vi "Control_Loop_Main.vi"(8 "error in (no error)":errorcluster) -> (0 "error out":errorcluster, 2 "loop":i32, 3 "pkg recived":timestamp)   [LabVIEW 2019, in "Service.lvlib"]
uses:
  Service.lvlib
  TypeDef/Control_loop_states.ctl
  TypeDef/AppData.ctl
  MsgQ/TypeDefs/CommandsQ.ctl
  MsgQ/TypeDefs/MsgQ_Commands.ctl
  zmq_multipart_lib/src_LabVIEW/zmq_mulipart_lib/zmq_multipart_lib.lvclass
  <vilib>/Field R&D Services/Logger/Type Definitions/Severity.ctl
  <vilib>/Field R&D Services/Logger/Support/Manager.vi
  <vilib>/Field R&D Services/Logger/Field_RnD_Services_Logger_Toolkit.lvlib
  mmw_command_lib/src_LabVIEW/mmW_commands/mmW_commands.lvlib
  MsgQ/MsgQ.lvlib
panel:
  out "status":T1
  out "data DVR out":refnum<data-value>
  out "Mode":enum16{"RF", "IF", "BB"}(ring)
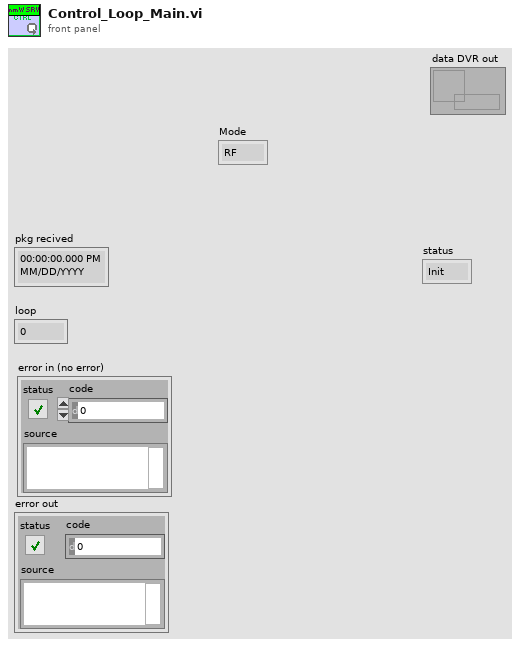
[diagram p1: front panel]
types:
  T1 = typedef "Service.lvlib/Control_loop_states.ctl" = enum16{"Init", "Create_listener", "Read", "Waiting_for_UI", "Send_response", "Close"}
  T2 = typedef "Service.lvlib/AppData.ctl" = cluster{"MsgQ":refnum<queue>, "Stop?":bool, "zmq sessions":cluster{"Control_endpoint":string, "Instr_endpoint":string}, "control-loop":cluster{"fromUI-Q":refnum<queue>, "toUI":refnum<user-event>, "Control_endpoint":string}, "UI-loop":cluster{"evnt_ref":refnum<event-registration>}, "logging":cluster{"level":dbl, "verbosity":dbl, "path":string, "Listener_ID":string}, "general_settings":cluster{"mmW_instr_ini_path":string, "mmW_instr_pid_path":string}}
  T3 = typedef "Field_RnD_Services_Logger_Toolkit.lvlib/Severity.ctl" = enum16{"Benign", "Warning", "Recoverable", "Fatal"}
  T4 = typedef "mmW_commands.lvlib/mode.ctl" = enum16{"RF", "IF", "BB"}
  T5 = typedef "mmW_commands.lvlib/commands.ctl" = enum16{"configure_fs", "configure_rf", "configure_trigger", "equalization_enable", "equalization_start", "lo_sync_enable", "equalization_stop", "get_instrument_status", "get_versions", "initialize_hw", "pop_rx", "set_log_level", "Shutdown", "start", "start_instrument_app", "stop", "trans", "transceive", "trigger_burst", "trigger_sync_enable", "Write TX", "resp_generic", "resp_waveform", "send_trigger", "fetch", "transceive2"}
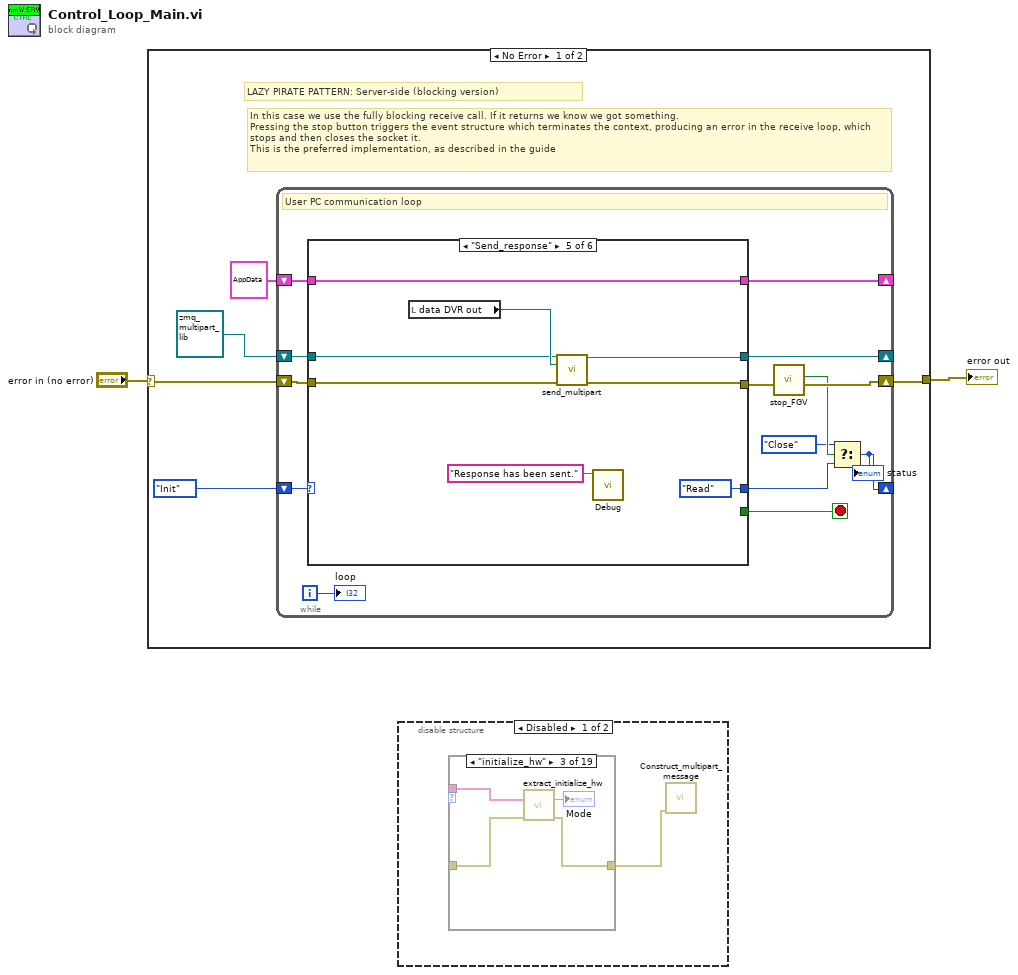
[diagram p0: block diagram]
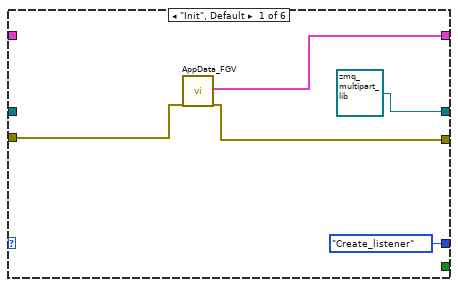
[diagram p2: hidden frame]
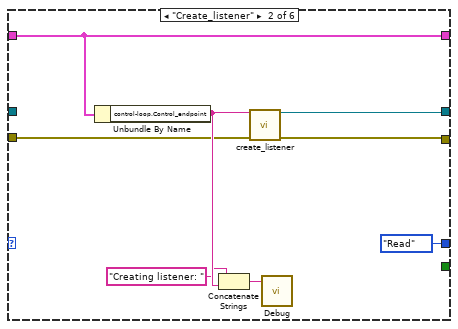
[diagram p3: hidden frame]
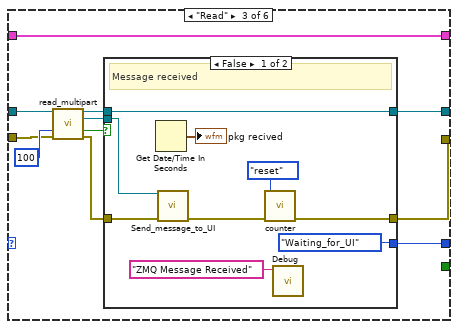
[diagram p4: hidden frame]
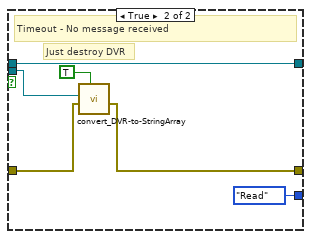
[diagram p5: hidden frame]
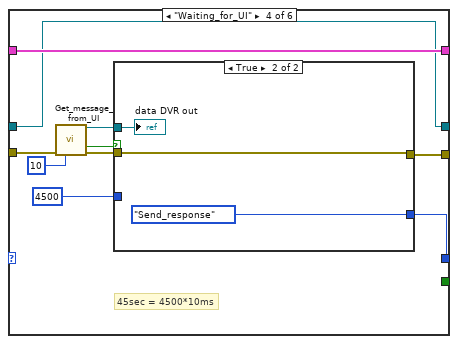
[diagram p6: hidden frame]
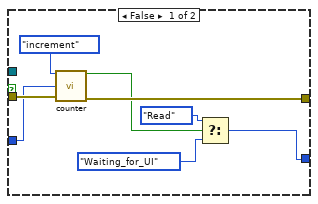
[diagram p7: hidden frame]
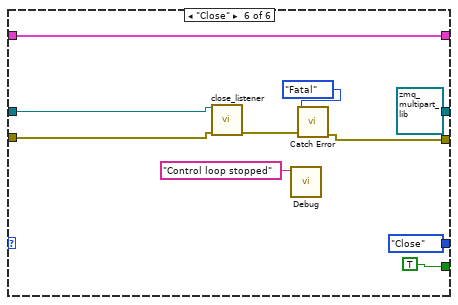
[diagram p8: hidden frame]
diagram:
  n1 = case shown="No Error" "error in (no error)" {
    selector: "error in (no error)" -> [w4 w100]
    tunnel: [w3 w100] -> w2
    frame No Error {
      # "In this case we use the fully blocking receive call. If it returns we know we got something.\nPressing the stop button triggers the event structure which terminates the context, producing an error in the receive loop, which stops and then closes the socket it.\nThis is the preferred implementation, as described in the guide"
      # "LAZY PIRATE PATTERN: Server-side (blocking version)"
      n2 = while {
        shift-right: [w19] -> w3
        shift-left: w4 -> [w17]
        shift-right: [w9] -> _
        shift-left: Control_loop_states."Init" -> [w15]
        shift-right: [w14] -> _
        shift-left: T2 {"MsgQ"=refnum, "Stop?"=FALSE, "zmq sessions"={"Control_endpoint"="", "Instr_endpoint"=""}, "control-loop"={"fromUI-Q"=refnum, "toUI"=refnum, "Control_endpoint"=""}, "UI-loop"={"evnt_ref"=refnum}, "logging"={"level"=0.0, "verbosity"=0.0, "path"="", "Listener_ID"=""}, "general_settings"={"mmW_instr_ini_path"="", "mmW_instr_pid_path"=""}} ("AppData out") -> [w13]
        shift-right: [w16] -> _
        shift-left: refnum<class "zmq_multipart_lib.lvclass"> refnum ("zmq_mlt out") -> [w18]
        i -> [w21]
        stop <- w12 stop-if-true
        # "User PC communication loop"
        n3 = case shown="\"Send_response\"" w15 {
          tunnel: [w24 w28 w45 w63 w84 w92] -> w20
          tunnel: w18 -> [_ _ w44 w61 w87 w90]
          tunnel: w17 -> [w25 w30 w42 w69 w85 w91]
          tunnel: [refnum<class "zmq_multipart_lib.lvclass"> refnum ("zmq_mlt out") w31 w37 w61 w86 refnum<class "zmq_multipart_lib.lvclass"> refnum ("zmq_mlt out")] -> w16
          tunnel: [w26 w29 w36 w70 w89 w99] -> w14
          tunnel: w13 -> [_ w29 w36 w70 w89 w99]
          tunnel: [Control_loop_states."Create_listener" Control_loop_states."Read" w35 w65 Control_loop_states."Read" Control_loop_states."Close"] -> w10
          tunnel: [_ _ _ _ _ TRUE] -> w12
          frame "Init", Default {
            n4 = call "AppData_FGV.vi"("error in (no error)"=w25) -> ("AppData out"=w26:T2, "error out"=w24:errorcluster)  [unwired: 17 in]
          }
          frame "Create_listener" {
            n5 = Unbundle By Name(w29) -> ("control-loop.Control_endpoint"=w34:string)
            n6 = Concatenate Strings("Creating listener: " ("string"), w34) -> (w33:string)
            n7 = call "create_listener.vi"("control_endpoint"=w34, "error in (no error)"=w30) -> ("zmq_mlt out"=w31:refnum<class "zmq_multipart_lib.lvclass">, "error out"=w28:errorcluster)  [unwired: 12 in]
            n8 = call <vilib>:"Debug.vi"("Message"=w33) -> ()  [unwired: 10 in, 1 out]
          }
          frame "Read" {
            n9 = call "read_multipart.vi"("zmq_mlt in"=w44, "timeout (ms)"=u32 100, "error in (no error)"=w42) -> ("zmq_mlt out"=w38:refnum<class "zmq_multipart_lib.lvclass">, "multipart message DVR"=w41:refnum<data-value>, "timeout?"=w40:bool, "error out"=w39:errorcluster)  [unwired: 8 in, 1 out]
            n10 = case shown="False" w40 {
              tunnel: w41 -> [w52 w59]
              tunnel: w39 -> [w51 w58]
              tunnel: [w46 w57] -> w45
              tunnel: w38 -> [w49 w60]
              tunnel: [w49 w60] -> w37
              tunnel: [Control_loop_states."Waiting_for_UI" Control_loop_states."Read"] -> w35
              frame False {
                # "Message received"
                n11 = Get Date/Time In Seconds() -> (seconds since 1Jan1904=→"pkg recived":timestamp)
                n12 = call "Send_message_to_UI.vi"("Data Value Reference in"=w52, "error in (no error)"=w51) -> ("error out"=w47:errorcluster)  [unwired: 13 in]
                n13 = call "counter.vi"("mode"=enum16{"increment", "decrement", "reset"}."reset", "error in (no error)"=w47) -> ("error out"=w46:errorcluster)  [unwired: 12 in, 1 out]
                n14 = call <vilib>:"Debug.vi"("Message"="ZMQ Message Received") -> ()  [unwired: 10 in, 1 out]
              }
              frame True {
                # "Just destroy DVR"
                # "Timeout - No message received"
                n15 = call "convert_DVR-to-StringArray.vi"("Delete DVR? (T)"=TRUE, "error in (no error)"=w58, "multipart message DVR in"=w59) -> ("error out"=w57:errorcluster)  [unwired: 5 in, 1 out]
              }
            }
          }
          frame "Waiting_for_UI" {
            # "45sec = 4500*10ms"
            n16 = call "Get_message_from_UI.vi"("error in (no error)"=w69, "timeout in ms (1000)"=10) -> ("data DVR out"=w68:refnum<data-value>, "output valid?"=w66:bool, "error out"=w64:errorcluster)  [unwired: 11 in]
            n17 = case shown="True" w66 {
              tunnel: w68 -> [_ w81]
              tunnel: [w71 Control_loop_states."Send_response"] -> w65
              tunnel: w64 -> [w78 w79]
              tunnel: [w77 w79] -> w63
              tunnel: 4500 -> [w75 _]
              frame False {
                n18 = call "counter.vi"("mode"=enum16{"increment", "decrement", "reset"}."increment", "limit"=w75, "error in (no error)"=w78) -> ("limit reached?"=w74:bool, "error out"=w77:errorcluster)  [unwired: 11 in]
                n19 = Select(t=Control_loop_states."Read", s=w74, f=Control_loop_states."Waiting_for_UI") -> (s? t:f=w71:T1)
              }
              frame True {
                "data DVR out" <- w81
              }
            }
          }
          frame "Send_response" {
            n20 = local read "data DVR out"() -> (w88:refnum<data-value>)
            n21 = call "send_multipart.vi"("zmq_mlt in"=w87, "multipart mesage in"=w88, "error in (no error)"=w85) -> ("zmq_mlt out"=w86:refnum<class "zmq_multipart_lib.lvclass">, "error out"=w84:errorcluster)  [unwired: 11 in]
            n22 = call <vilib>:"Debug.vi"("Message"="Response has been sent.") -> ()  [unwired: 10 in, 1 out]
          }
          frame "Close" {
            n23 = call "close_listener.vi"("zmq_mlt in"=w90, "error in (no error)"=w91) -> ("error out"=w93:errorcluster)  [unwired: 12 in, 1 out]
            n24 = call <vilib>:"Debug.vi"("Message"="Control loop stopped") -> ()  [unwired: 10 in, 1 out]
            n25 = call <vilib>:"Catch Error.vi"("Error In"=w93, "Severity"=Severity."Fatal") -> ("Error Out"=w92:errorcluster)  [unwired: 9 in]
          }
        }
        n26 = call "stop_FGV"("error in (no error)"=w20) -> ("error out"=w19:errorcluster, "stop?"=w11:bool)  [unwired: 7 in]
        n27 = Select(t=Control_loop_states."Close", s=w11, f=w10) -> (s? t:f=w9:T1)
        "status" <- w9
        "loop" <- w21
      }
    }
    frame Error {
    }
  }
  "error out" <- w2
  n28 = disable-structure shown="Disabled" {
    frame Disabled {
      n29 = case shown="\"initialize_hw\"" {
        selector: _ -> [_ _ _ _ _ _ _ _ _ _ _ _ _ _ _ _ _ _ _]
        tunnel: _ -> [_ _ w108 _ _ _ _ _ _ _ _ _ _ _ _ _ _ w123 _]
        tunnel: _ -> [w103 w104 w107 w109 w110 w111 w112 w113 w114 w115 w116 w117 w118 w119 w120 w121 w122 w125 w126]
        tunnel: [w103 w104 w106 w109 w110 w111 w112 w113 w114 w115 w116 w117 w118 w119 w120 w121 w122 w124 w126] -> w101
        frame "configure_rf", Default {
        }
        frame "configure_trigger" {
        }
        frame "initialize_hw" {
          n30 = call "extract_initialize_hw.vi"("multipart message in"=w108, "error in (no error)"=w107) -> ("Mode"=→"Mode":T4, "error out"=w106:errorcluster)  [unwired: 9 in, 3 out]
        }
        frame "pop_rx" {
        }
        frame "lo_sync_enable" {
        }
        frame "equalization_stop" {
        }
        frame "start" {
        }
        frame "stop" {
        }
        frame "trigger_burst" {
        }
        frame "Shutdown" {
        }
        frame "transceive" {
        }
        frame "resp_generic" {
        }
        frame "resp_waveform" {
        }
        frame "equalization_enable" {
        }
        frame "equalization_start" {
        }
        frame "set_log_level" {
        }
        frame "trigger_sync_enable" {
        }
        frame "Write TX" {
          n31 = call "extract_Write Tx.vi"("multipart message in"=w123, "error in (no error)"=w125) -> ("error out"=w124:errorcluster)  [unwired: 8 in, 5 out]
        }
        frame "configure_fs" {
        }
      }
      n32 = call "Construct_multipart_message.vi"("error in (no error)"=w101) -> ("command"=w102:T5)  [unwired: 10 in, 4 out]
    }
    frame Enabled {
    }
  }
